vi "save_data_test.vi"() -> ()   [LabVIEW 2013]
panel:
  in  "seconds  to wait":u32
  out "Median FITC/SSC":dbl(graph)
  out "Median":dbl format="%0.2f"
  in  "stop":bool
  in  "LED CONTROLS":dbl[][](array[numeric])
  in  "error in":errorcluster
  in  "DIVA DIRECTORY":path=path "D:/BDDatabase/BDData"
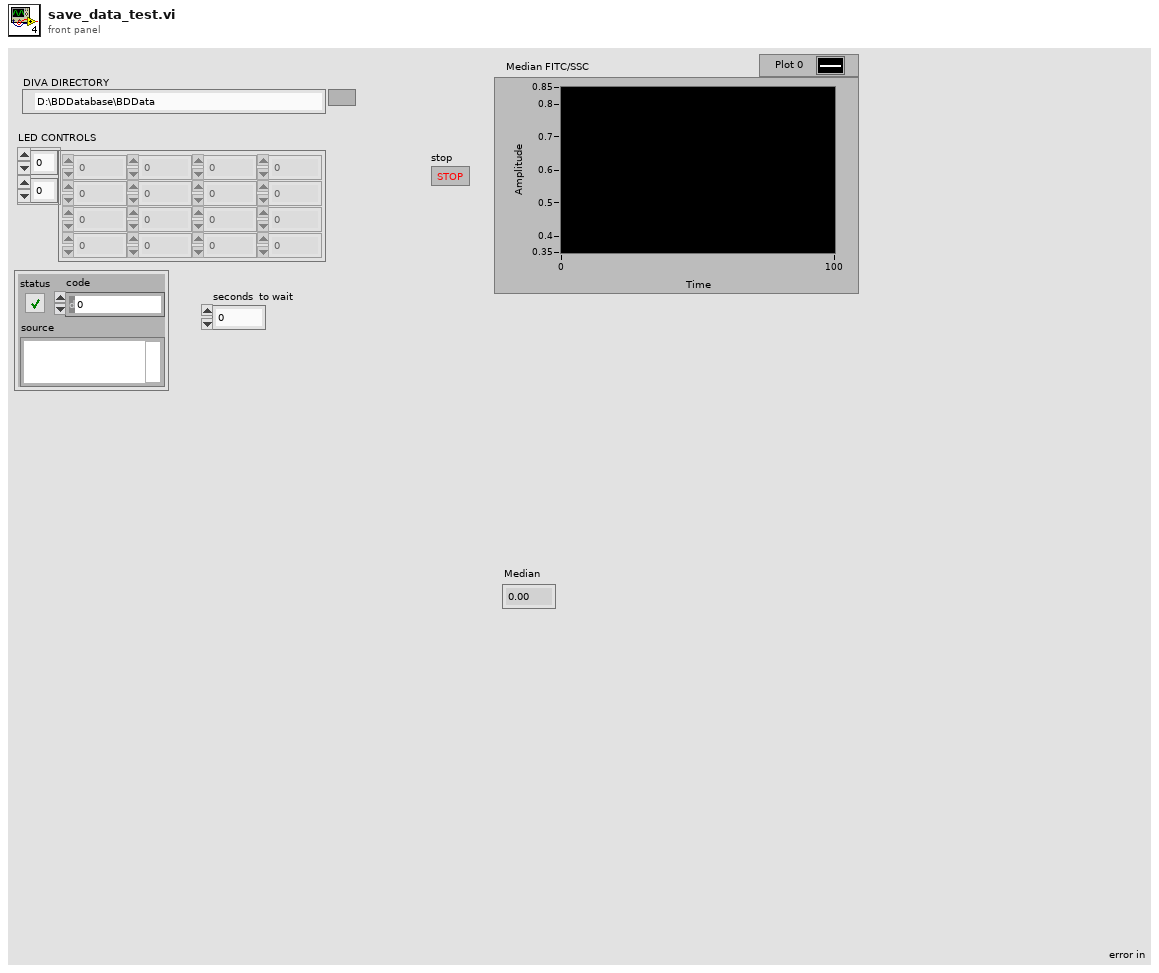
[diagram p1: front panel]
types:
  T1 = cluster{i32, "LED CONTROLS":dbl[], "TIME STAMPS":dbl[], "LAST MEASUREMENT":dbl[][], "SUMMARY STAT":dbl[]}[]
  T2 = cluster{i32, "LED CONTROLS":dbl[], "TIME STAMPS":dbl[], "LAST MEASUREMENT":dbl[][], "SUMMARY STAT":dbl[]}
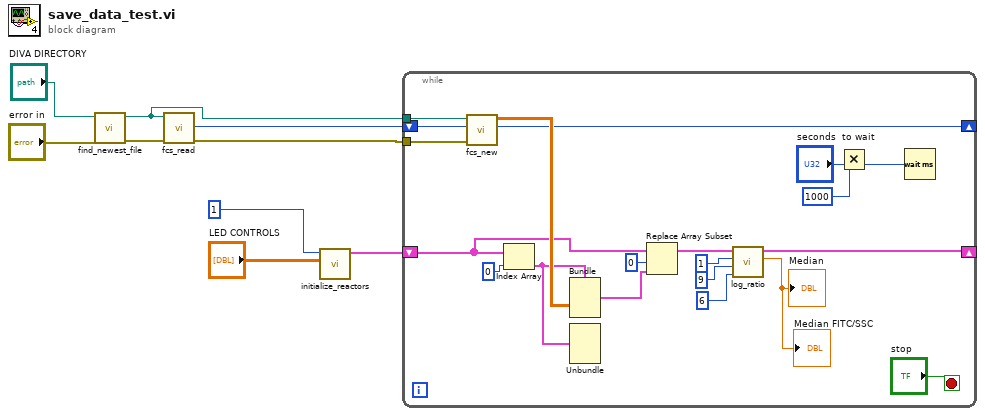
[diagram p0: block diagram]
diagram:
  n1 = call "find_newest_file.vi"("error in"="error in", "Directory Path to Start the Search"="DIVA DIRECTORY") -> ("error out"=w7:errorcluster, "Most Recent File Path"=w4:path)  [unwired: 6 in, 1 out]
  n2 = call "fcs_read.vi"("error in (no error)"=w7, "Path"=w4) -> ("error out"=w2:errorcluster, "byte offset"=w3:i64)  [unwired: 6 in, 2 out]
  n3 = call "initialize_reactors.vi"("LED CONTROLS"="LED CONTROLS", "Number of Reactors"=u32 1) -> ("REACTORS"=w1:T1)  [unwired: 9 in]
  n4 = while {
    tunnel: w4 -> [w28]
    tunnel: w2 -> [w26]
    shift-right: [w14] -> _
    shift-left: w3 -> [w27]
    shift-right: [w15] -> _
    shift-left: w1 -> [w22]
    stop <- "stop" stop-if-true
    n5 = call "fcs_new.vi"("error in (no error)"=w26, "byte offset in"=w27, "Path in"=w28) -> ("byte offset out"=w14:i64, "new data"=w24:sgl[][])  [unwired: 6 in, 1 out]
    n6 = Index Array(array=w22, index=0) -> (element=w23:T2)
    n7 = Bundle(cluster=w23, "LAST MEASUREMENT"=w24) -> (w21:T2)  [unwired: 4 in]
    n8 = Unbundle(w23) -> ()  [unwired: 5 out]
    n9 = Replace Array Subset(array=w22, new element=w21, index=0) -> (w19:T1)
    n10 = call "log_ratio.vi"("Y"=6, "X"=9, "Reactor"=1, "REACTORS"=w19) -> ("Median"=→"Median" →"Median FITC/SSC":dbl, "UPDATED REACTORS"=w15:T1)  [unwired: 6 in]
    n11 = Multiply(x=u32 1000, y="seconds  to wait") -> (x*y=w11:u32)
    n12 = Wait (ms)(milliseconds to wait=w11) -> ()  [unwired: 1 out]
  }
